vi "CC WebRelay Control.vi"(7 "Action":T1, 8 "error in (no error)":errorcluster, 10 "state":bool, 11 "Relay (1 to 10)":i32=1 min=1 max=10 step=1) -> (0 "error out":errorcluster, 3 "status":bool[](array[boolean]))   [LabVIEW 2024]
uses:
  CC WebRelay enum Actions.ctl
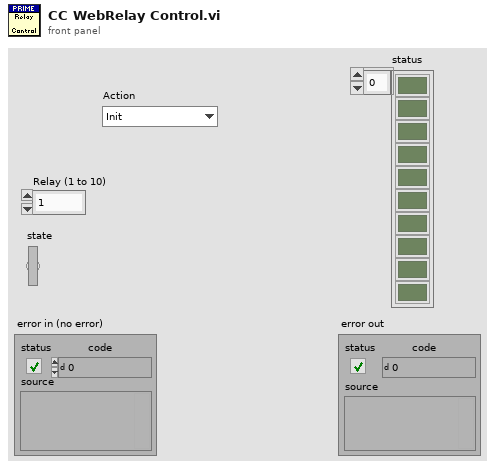
[diagram p1: front panel]
types:
  T1 = typedef "CC WebRelay enum Actions.ctl" = enum16{"Init", "Read Status", "Set Relay", "Close"}
  T2 = typedef "CC WebRelay cluster Settings.ctl" = cluster{"Address":string, "Port":u16, "Names":string[]}
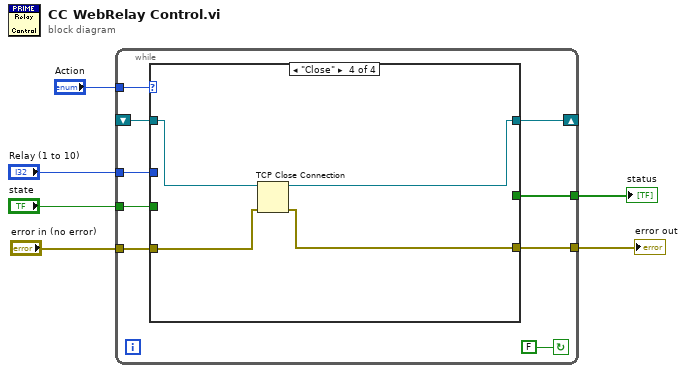
[diagram p0: block diagram]
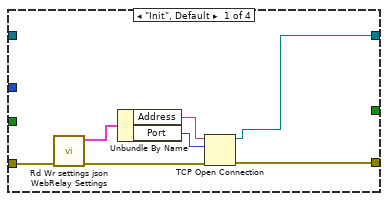
[diagram p2: hidden frame]
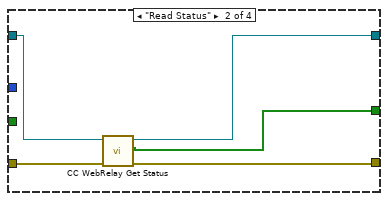
[diagram p3: hidden frame]
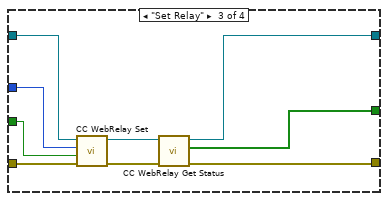
[diagram p4: hidden frame]
diagram:
  n1 = while {
    tunnel: "Action" -> [w15]
    tunnel: "error in (no error)" -> [w13]
    shift-right: [w12] -> _
    shift-left: _ -> [w11]
    tunnel: [w10] -> w4
    tunnel: [w9] -> w3
    tunnel: "Relay (1 to 10)" -> [w8]
    tunnel: "state" -> [w7]
    stop <- FALSE continue-if-true
    n2 = case shown="\"Close\"" w15 {
      tunnel: w13 -> [w21 w27 w36 w39]
      tunnel: [w17 w23 w29 w38] -> w12
      tunnel: w11 -> [_ w26 w35 w40]
      tunnel: [w16 w24 w30 w37] -> w10
      tunnel: [_ w25 w28 _] -> w9
      tunnel: w8 -> [_ _ w34 _]
      tunnel: w7 -> [_ _ w33 _]
      frame "Init", Default {
        n3 = call "Rd Wr settings json WebRelay Settings.vi"("error in (no error)"=w21) -> ("error out"=w20:errorcluster, "WebRelay10 Settings"=w22:T2)  [unwired: 9 in]
        n4 = Unbundle By Name(w22) -> ("Address"=w19:string, "Port"=w18:u16)
        n5 = TCP Open Connection(address=w19, remote port or service name=w18, error in (no error)=w20) -> (connection ID=w17:refnum<k5>, error out=w16:errorcluster)  [unwired: 2 in]
      }
      frame "Read Status" {
        n6 = call "CC WebRelay Get Status.vi"("error in (no error)"=w27, "connection ID"=w26) -> ("error out"=w24:errorcluster, "status"=w25:bool[], "connection ID out"=w23:refnum<k5>)  [unwired: 7 in]
      }
      frame "Set Relay" {
        n7 = call "CC WebRelay Set.vi"("error in (no error)"=w36, "state"=w33, "Relay (1 to 10)"=w34, "connection ID"=w35) -> ("error out"=w32:errorcluster, "connection ID out"=w31:refnum<k5>)  [unwired: 6 in]
        n8 = call "CC WebRelay Get Status.vi"("error in (no error)"=w32, "connection ID"=w31) -> ("error out"=w30:errorcluster, "status"=w28:bool[], "connection ID out"=w29:refnum<k5>)  [unwired: 7 in]
      }
      frame "Close" {
        n9 = TCP Close Connection(connection ID=w40, error in (no error)=w39) -> (connection ID out=w38:refnum<k5>, error out=w37:errorcluster)  [unwired: 1 in]
      }
    }
  }
  "error out" <- w4
  "status" <- w3
